vi "SelfTerminate.vi"(8 "error in (no error)":errorcluster, 11 "SMO in":refnum<class "SMO.lvclass">) -> (0 "error out":errorcluster, 3 "SMO out":refnum<class "SMO.lvclass">)   [LabVIEW 2021, in "smo.lvlib" / "SMO.lvclass"]
uses:
  SMO.lvclass
  SMO.lvclass/SMO.ctl
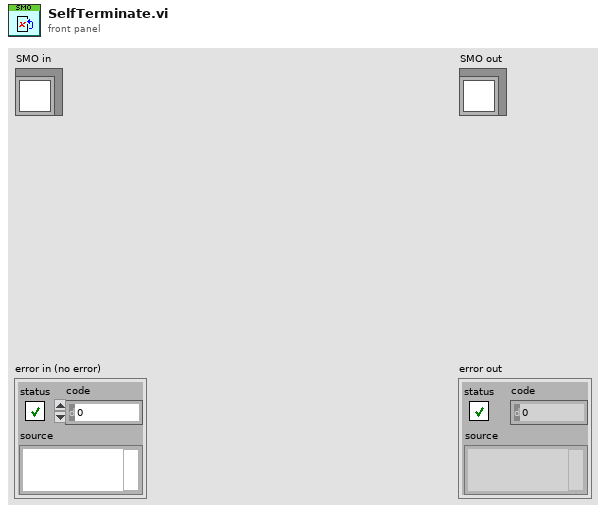
[diagram p1: front panel]
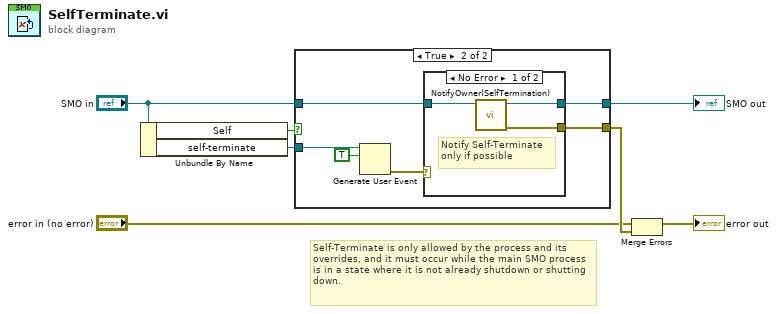
[diagram p0: block diagram]
diagram:
  # "Self-Terminate is only allowed by the process and its overrides, and it must occur while the main SMO process is in a state where it is not already shutdown or shutting down."
  n1 = Unbundle By Name("SMO in") -> ("Self"=w7:bool, "self-terminate"=w1:refnum<user-event>)
  n2 = case shown="True" w7 {
    tunnel: "SMO in" -> [w8 w10]
    tunnel: [w8 w14] -> w5
    tunnel: [_ w13] -> w4
    tunnel: w1 -> [_ w12]
    frame False {
    }
    frame True {
      n3 = Generate User Event(user event=w12, event data cluster=TRUE ("event data")) -> (error out=w9:errorcluster)  [unwired: 2 in, 1 out]
      n4 = case shown="No Error" w9 {
        tunnel: [w17 w18] -> w14
        tunnel: [w16 _] -> w13
        tunnel: w10 -> [w15 w18]
        frame No Error {
          # "Notify Self-Terminate\nonly if possible"
          n5 = call "NotifyOwner(SelfTermination).vi"("SMO in"=w15) -> ("error out"=w16:errorcluster, "SMO out"=w17:refnum<class "SMO.lvclass">)  [unwired: 9 in]
        }
        frame Error {
        }
      }
    }
  }
  "SMO out" <- w5
  n6 = Merge Errors("error in (no error)", w4) -> (→"error out":errorcluster)
